vi "Lockin raw points to average.vi"(9 "Lock-in settings":T2 {"Averaging period, s" format="%#_6p"}, 10 "CH name                          points   phase":T1, 11 "dt":dbl) -> (3 "Lockin raw points to average":i32)   [LabVIEW 2015]
uses:
  Syncronous Lockin Settings.ctl
  CH_name_pts_phase.ctl
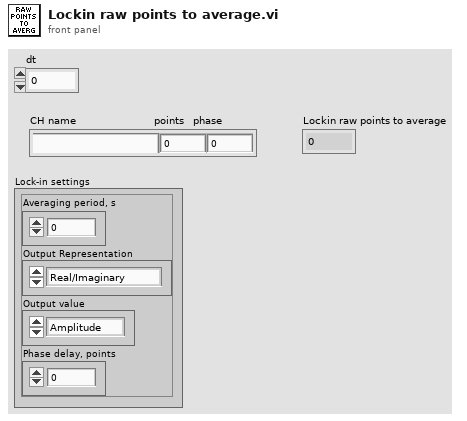
[diagram p1: front panel]
types:
  T1 = typedef "CH_name_pts_phase.ctl" = cluster{"Channel":string, "pts per sine wave":i32, "Phase":dbl}
  T2 = typedef "Syncronous Lockin Settings.ctl" = cluster{"Averaging period, s":dbl, "Output Representation":enum16{"Real/Imaginary", "Polar"}, "Output value":enum16{"Amplitude", "RMS", "Peak-to-Peak"}, "Phase delay, points":i32}
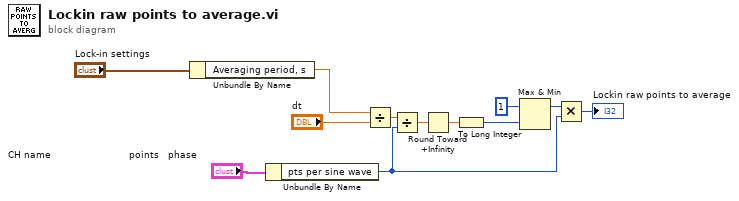
[diagram p0: block diagram]
diagram:
  n1 = Unbundle By Name("Lock-in settings") -> ("Averaging period, s"=w3:dbl)
  n2 = Unbundle By Name("CH name                          points   phase") -> ("pts per sine wave"=w11:i32)
  n3 = Divide(x=w3, y="dt") -> (x/y=w2:dbl)
  n4 = Divide(x=w2, y=w11) -> (x/y=w7:dbl)
  n5 = Round Toward +Infinity(x=w7) -> (ceil(x): smallest int >= x=w8:dbl)
  n6 = To Long Integer(number=w8) -> (32bit integer=w9:i32)
  n7 = Max & Min(x=1, y=w9) -> (max(x,y)=w1:i32)  [unwired: 1 out]
  n8 = Multiply(x=w1, y=w11) -> (x*y=→"Lockin raw points to average":i32)
